vi "Get Self Enqueuer.vi"(11 "eActor in":refnum<class "eActor.lvclass">) -> (2 "Actor Framework:Message Enqueuer":refnum<class "Message Enqueuer.lvclass">, 3 "eActor out":refnum<class "eActor.lvclass">)   [LabVIEW 2015, in "AMS UI.lvlib" / "eActor.lvclass"]
uses:
  eActor.lvclass
  <vilib>/ActorFramework/Message Enqueuer/Message Enqueuer.lvclass
  eActor.lvclass/eActor.ctl
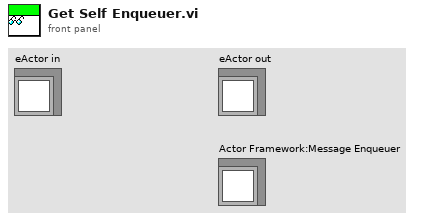
[diagram p1: front panel]
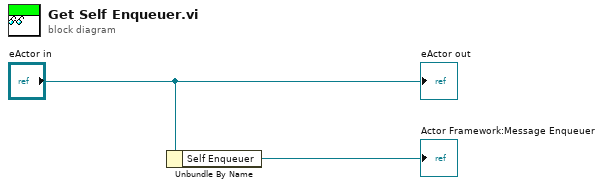
[diagram p0: block diagram]
diagram:
  n1 = Unbundle By Name("eActor in") -> ("Self Enqueuer"=→"Actor Framework:Message Enqueuer":refnum<class "Message Enqueuer.lvclass">)
  "eActor out" <- "eActor in"
